vi "West Arcade.vi"(4 "D Gain":dbl=5e-05 format="%#_13g", 6 "P Gain":dbl=0.0725 format="%#_13g", 8 "Operator":dbl, 9 "Buttons":bool[](array[boolean]), 10 "Axes":dbl[](array[numeric]), 11 "Get All":T2 {"Calibration"."CurrentMode" items=["BootTareGryoAccel"=0, "Temperature"=1, "Magnetometer12Pt"=2, "Magnetometer360"=3, "Accelerometer"=5]}) -> (2 "Left Motor Value":dbl, 3 "Right Motor Value":dbl, 5 "Control Mode":T1)   [LabVIEW 2016]
doc: "Employs the operations of the spin ez VI and the drive stright pigeon VI using the Joystick to dial and omnidirectional throttle VI.\n\nCreated by Team 4130 for use in the 2016-2017 FRC season"
uses:
  <vilib>/Rock Robotics/WPI/ThirdParty/Sensors/Pigeon IMU/CTRE_PigeonIMU_GlobalStatus.ctl
  <vilib>/Rock Robotics/WPI/ThirdParty/Sensors/Pigeon IMU/CTRE_PigeonIMU_PigeonState.ctl
  <vilib>/Rock Robotics/WPI/ThirdParty/Sensors/Pigeon IMU/CTRE_PigeonIMU_CalibrationMode.ctl
  <vilib>/Rock Robotics/WPI/ThirdParty/CanMotor/TalonSRX/WPI_CANTalonSRX_APIControlMode.ctl
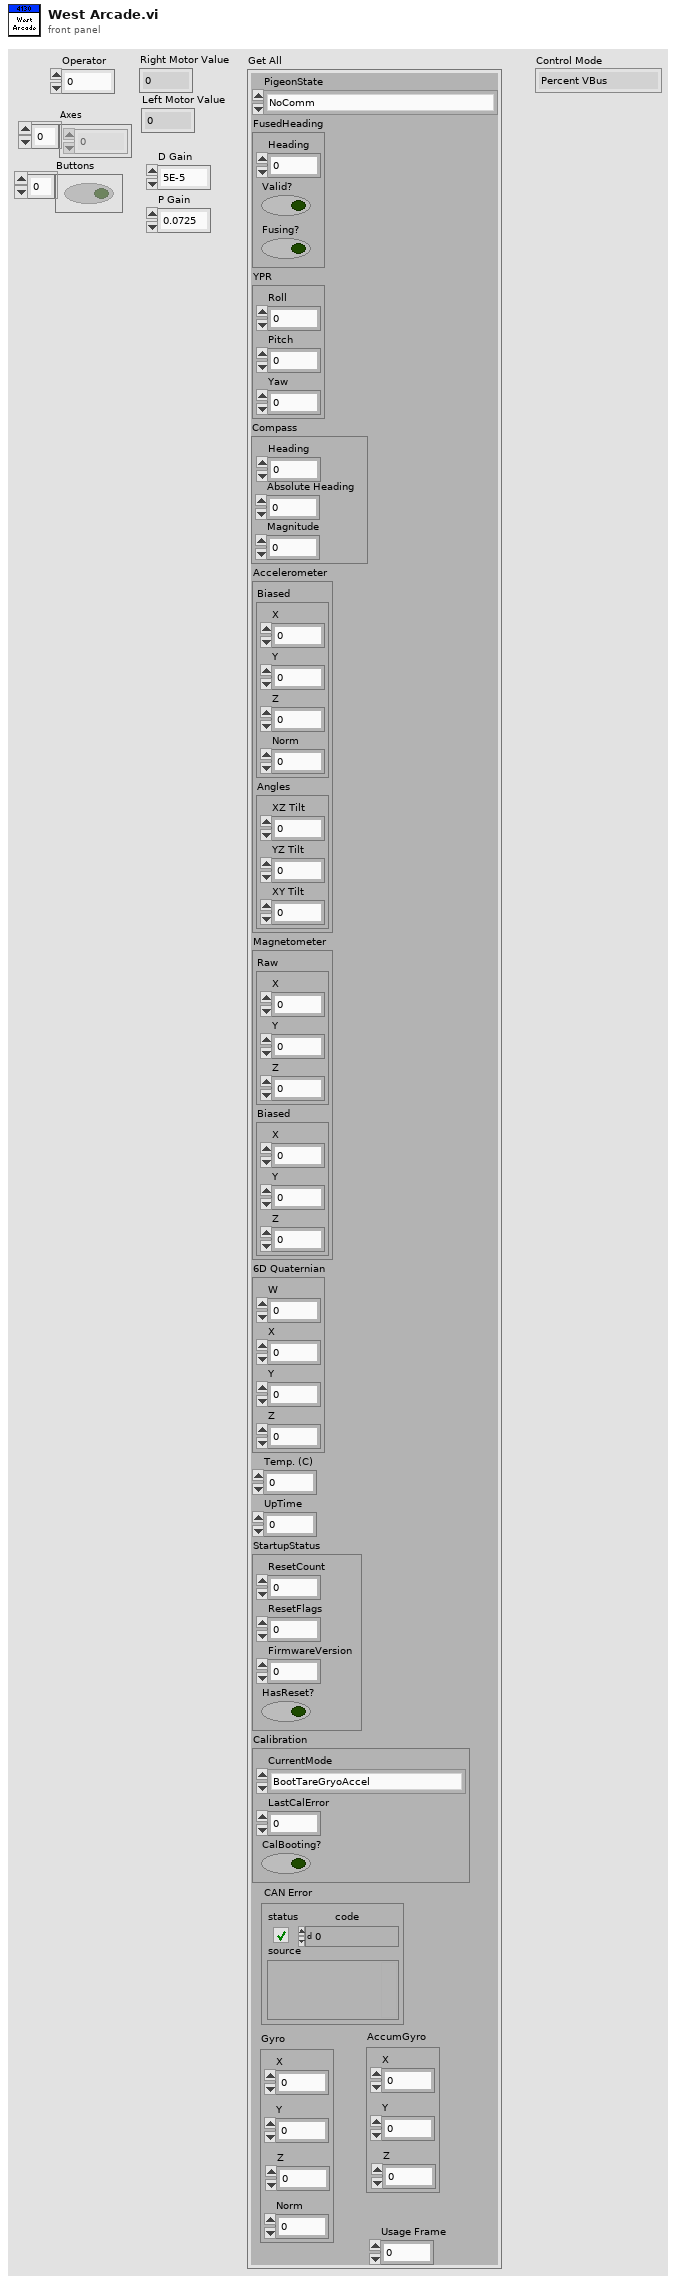
[diagram p1: front panel]
types:
  T1 = typedef "WPI_CANTalonSRX_APIControlMode.ctl" = enum8{"Percent VBus", "Speed", "Position", "Slave", "Unchanged / Invalid", "Voltage Compensation", "Current", "Motion Profile", "Motion Magic"}
  T2 = typedef "CTRE_PigeonIMU_GlobalStatus.ctl" = cluster{"PigeonState":T3, "FusedHeading":cluster{"Heading":dbl, "Valid?":bool, "Fusing?":bool}, "YPR":cluster{"Yaw":dbl, "Pitch":dbl, "Roll":dbl}, "Compass":cluster{"Heading":dbl, "Magnitude":dbl, "Absolute Heading":dbl}, "Accelerometer":cluster{"Biased":cluster{"X":i16, "Y":i16, "Z":i16, "Norm":i16}, "Angles":cluster{"XZ Tilt":dbl, "YZ Tilt":dbl, "XY Tilt":dbl}}, "Magnetometer":cluster{"Raw":cluster{"X":i16, "Y":i16, "Z":i16}, "Biased":cluster{"X":i16, "Y":i16, "Z":i16}}, "Gyro":cluster{"X":dbl, "Y":dbl, "Z":dbl, "Norm":dbl}, "6D Quaternian":cluster{"W":dbl, "X":dbl, "Y":dbl, "Z":dbl}, "Temp. (C)":dbl, "UpTime":u32, "StartupStatus":cluster{"ResetCount":i32, "ResetFlags":i32, "FirmwareVersion":i32, "HasReset?":bool}, "Calibration":cluster{"CurrentMode":T4, "LastCalError":i32, "CalBooting?":bool}, "CAN Error":errorcluster, "AccumGyro":cluster{"X":dbl, "Y":dbl, "Z":dbl}, "Usage Frame":u32}
  T3 = typedef "CTRE_PigeonIMU_PigeonState.ctl" = enum16{"NoComm", "Initializing", "Ready", "UserCalibration"}
  T4 = typedef "CTRE_PigeonIMU_CalibrationMode.ctl" = u16
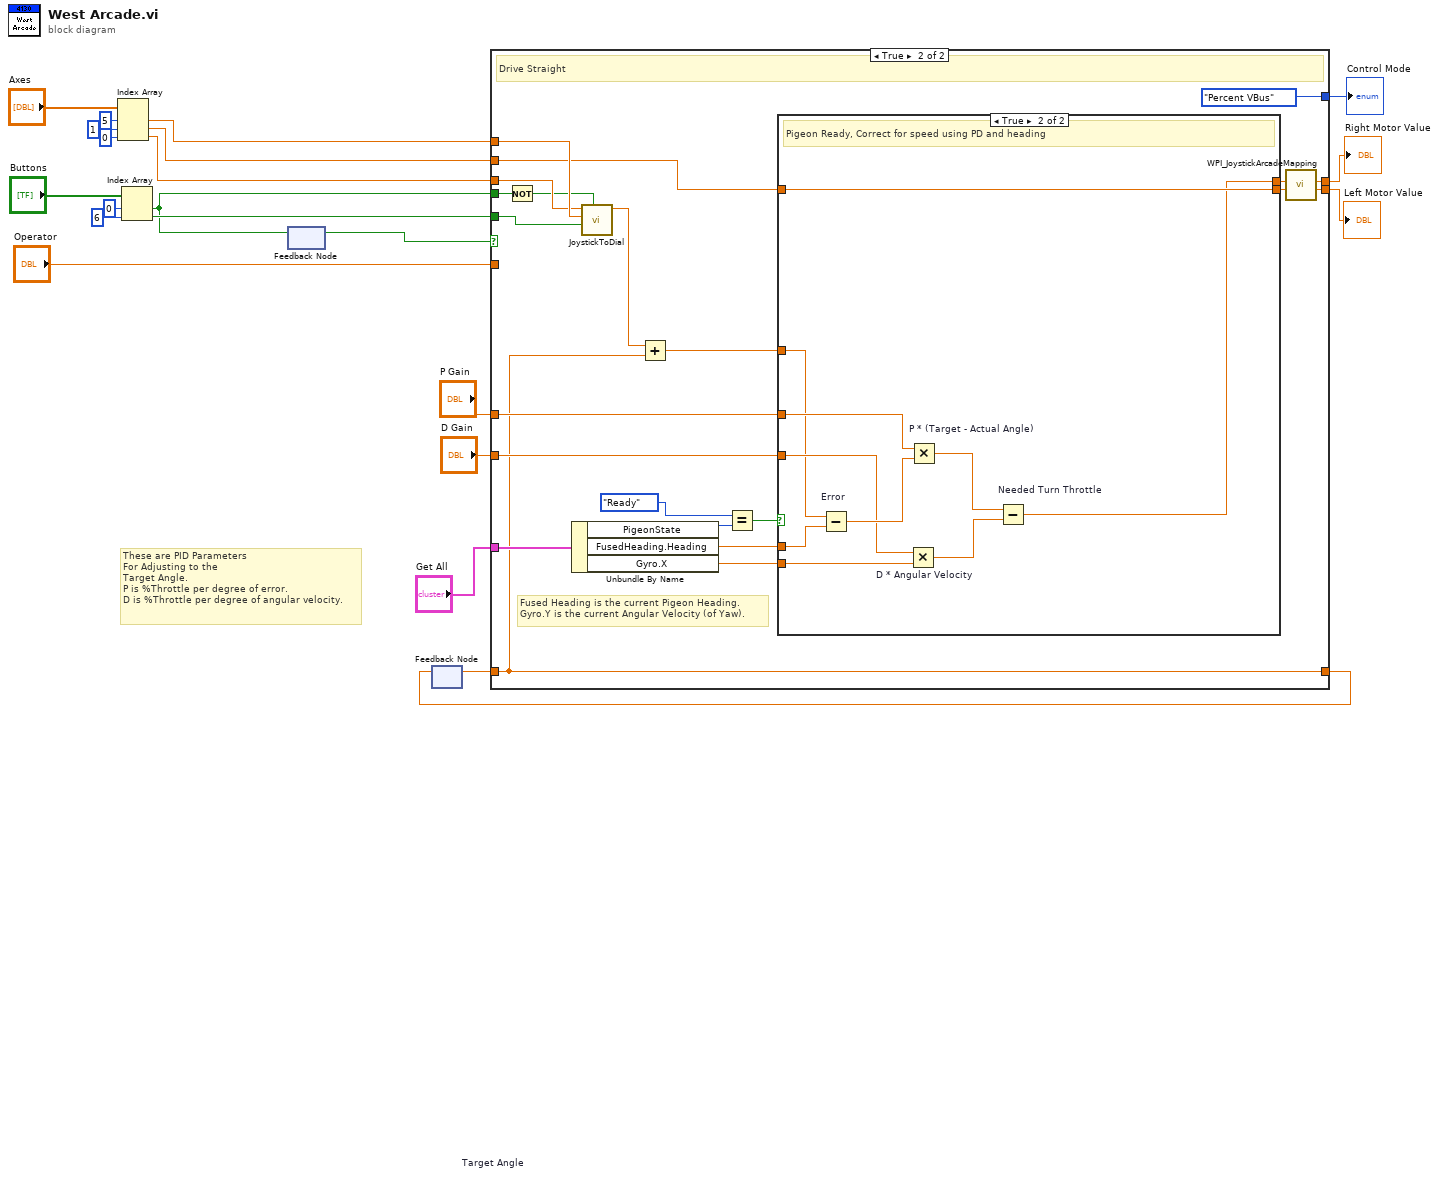
[diagram p0: block diagram]
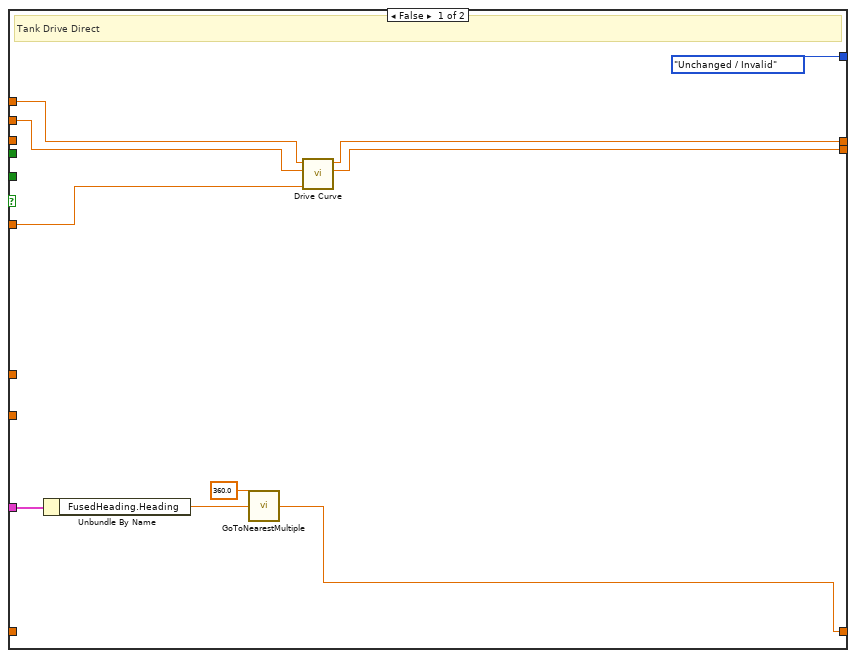
[diagram p2: hidden frame]
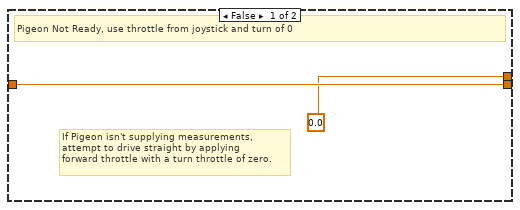
[diagram p3: hidden frame]
diagram:
  # "These are PID Parameters\nFor Adjusting to the\nTarget Angle.\nP is %Throttle per degree of error.\nD is %Throttle per degree of angular velocity."
  n1 = Index Array(array="Axes", index #1=5 ("index"), index #2=1 ("index"), index #3=0 ("index")) -> (element #1=w13:dbl, element #2=w12:dbl, element #3=w7:dbl)
  n2 = Index Array(array="Buttons", index #1=0 ("index"), index #2=6 ("index")) -> (element #1=w1:bool, element #2=w8:bool)
  n3 = feedback-in #1(w1) -> ()
  n4 = feedback #1() -> (w2:bool)  [unwired: 1 in]
  n5 = feedback #2 "Target Angle"() -> (w20:dbl)  [unwired: 1 in]
  n6 = case shown="True" w2 {
    tunnel: w13 -> [w31 w37]
    tunnel: w12 -> [w30 w36]
    tunnel: "P Gain" -> [_ w49]
    tunnel: "D Gain" -> [_ w48]
    tunnel: [w24 w40] -> w19
    tunnel: w20 -> [_ w40]
    tunnel: [w29 w45] -> w18
    tunnel: [w28 w44] -> w17
    tunnel: "Get All" -> [w32 w43]
    tunnel: "Operator" -> [w27 _]
    tunnel: [WPI_CANTalonSRX_APIControlMode."Unchanged / Invalid" ("Control Mode") WPI_CANTalonSRX_APIControlMode."Percent VBus" ("Control Mode")] -> w10
    tunnel: w8 -> [_ w38]
    tunnel: w7 -> [_ w35]
    tunnel: w1 -> [_ w33]
    frame False {
      # "Tank Drive Direct"
      n7 = Unbundle By Name(w32) -> ("FusedHeading.Heading"=w25:dbl)
      n8 = call "GoToNearestMultiple.vi"("Multiple"=360.0, "Numeric"=w25) -> ("Snapped Numeric"=w24:dbl)  [unwired: 13 in]
      n9 = call "Drive Curve.vi"("Operator"=w27, "Left"=w30, "Right"=w31) -> ("Left"=w28:dbl, "Right"=w29:dbl)  [unwired: 7 in]
    }
    frame True {
      # "Fused Heading is the current Pigeon Heading.\nGyro.Y is the current Angular Velocity (of Yaw)."
      # "Drive Straight"
      n10 = Not(x=w33) -> (.not. x?=w34:bool)
      n11 = Unbundle By Name(w43) -> ("PigeonState"=w52:T3, "FusedHeading.Heading"=w51:dbl, "Gyro.X"=w50:dbl)
      n12 = call "JoystickToDial.vi"("Reset"=w34, "Reverse"=w38, "Y"=w37, "X"=w35) -> ("Heading"=w41:dbl)  [unwired: 6 in, 1 out]
      n13 = Add(x=w41, y=w40) -> (x+y=w39:dbl)
      n14 = Equal?(x=CTRE_PigeonIMU_PigeonState."Ready" ("PigeonState"), y=w52) -> (x = y?=w54:bool)
      n15 = case shown="True" w54 {
        tunnel: w36 -> [w56 w59]
        tunnel: [w56 w59] -> w46
        tunnel: [0.0 ("upper limit") w57] -> w47
        tunnel: w51 -> [_ w66]
        tunnel: w39 -> [_ w58]
        tunnel: w50 -> [_ w63]
        tunnel: w49 -> [_ w64]
        tunnel: w48 -> [_ w62]
        frame False {
          # "If Pigeon isn't supplying measurements,\nattempt to drive straight by applying\nforward throttle with a turn throttle of zero."
          # "Pigeon Not Ready, use throttle from joystick and turn of 0"
        }
        frame True {
          # "Pigeon Ready, Correct for speed using PD and heading"
          n16 = Subtract "Error"(x=w58, y=w66) -> (x-y=w65:dbl)
          n17 = Multiply "D * Angular Velocity"(x=w62, y=w63) -> (x*y=w60:dbl)
          n18 = Multiply "P * (Target - Actual Angle)"(x=w64, y=w65) -> (x*y=w61:dbl)
          n19 = Subtract "Needed Turn Throttle"(x=w61, y=w60) -> (x-y=w57:dbl)
        }
      }
      n20 = call <vilib>:"WPI_JoystickArcadeMapping.vi"("Y axis value"=w46, "X axis value"=w47) -> ("Right Motor Value"=w44:dbl, "Left Motor Value"=w45:dbl)  [unwired: 8 in]
    }
  }
  "Right Motor Value" <- w18
  "Left Motor Value" <- w17
  "Control Mode" <- w10
  n21 = feedback-in #2(w19) -> ()
